vi "Change Selection.vi"(8 "error in (no error)":errorcluster, 10 "Coords":T1, 11 "PieChart in":refnum<class "PieChart.lvclass">) -> (0 "error out":errorcluster, 3 "PieChart out":refnum<class "PieChart.lvclass">)   [LabVIEW 2018, in "PieChart.lvclass"]
uses:
  PieChart.lvclass
  <vilib>/Utility/miscctls.llb/LVPoint32TypeDef.ctl
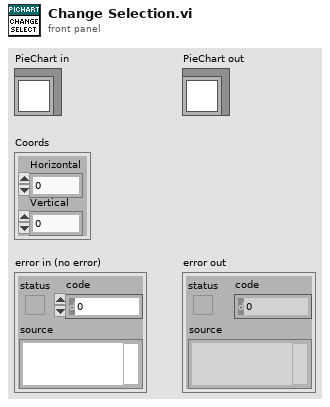
[diagram p1: front panel]
types:
  T1 = typedef "LVPoint32TypeDef.ctl" = cluster{"Horizontal":i32, "Vertical":i32}
  T2 = typedef "PieChart.lvclass/Pie info for Click.ctl" = cluster{"Slice Positions":cluster{"Start":i16, "End":i16}[], "Center Position":T3, "Radius":i16}
  T3 = typedef "LVBoundsTypeDef.ctl" = cluster{"Width":u32, "Height":u32}
  T4 = typedef "LVRectTypeDef.ctl" = cluster{"Left":i16, "Top":i16, "Right":i16, "Bottom":i16}
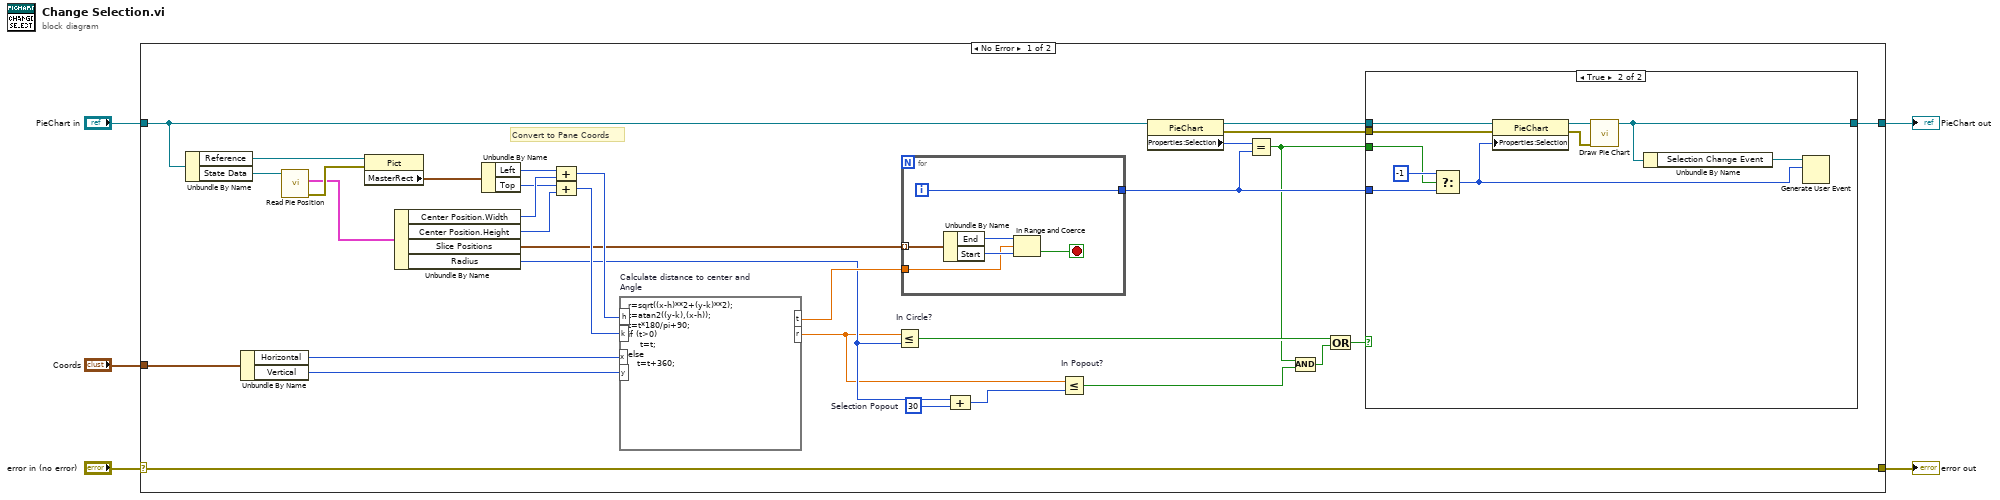
[diagram p0: block diagram]
diagram:
  n1 = case shown="No Error" "error in (no error)" {
    selector: "error in (no error)" -> [w37 w56]
    tunnel: [w37 w56] -> w4
    tunnel: [w20 w55] -> w2
    tunnel: "PieChart in" -> [w9 w55]
    tunnel: "Coords" -> [w27 _]
    frame No Error {
      w19 = i16 30  # Selection Popout
      # "Convert to Pane Coords"
      n2 = Unbundle By Name(w9) -> ("Reference"=w35:refnum<vi>, "State Data"=w36:refnum<data-value>)
      n3 = Unbundle By Name(w27) -> ("Horizontal"=w26:i32, "Vertical"=w25:i32)
      n4 = call "Read Pie Position.vi"("Data Value Reference in"=w36) -> ("error out"=w33:errorcluster, "Slice Positions"=w28:T2)  [unwired: 9 in]
      n5 = property class="Pict"(reference=w35, error in=w33) -> ("MasterRect"=w34:T4)  [unwired: 2 out]
      n6 = Unbundle By Name(w28) -> ("Center Position.Width"=w31:u32, "Center Position.Height"=w29:u32, "Slice Positions"=w6:cluster{"Start":i16, "End":i16}[], "Radius"=w18:i16)
      n7 = Unbundle By Name(w34) -> ("Left"=w32:i16, "Top"=w30:i16)
      n8 = Compound Arithmetic op=ADD(w32, w31) -> (w24:u32)
      n9 = Compound Arithmetic op=ADD(w30, w29) -> (w23:u32)
      n10 = formula code="r=sqrt((x-h)**2+(y-k)**2);\nt=atan2((y-k),(x-h));\nt=t*180/pi+90;\nif (t>0)\n    t=t;\nelse\n   t=t+360;" "Calculate distance to center and\nAngle"("x"=w26, "y"=w25, "h"=w24, "k"=w23) -> ("r"=w17:dbl, "t"=w22:dbl)
      n11 = Less Or Equal? "In Circle?"(x=w17, y=w18) -> (x <= y?=w15:bool)
      n12 = for {
        tunnel: w6 -> [w54] mode=indexing
        tunnel: w22 -> [w51]
        tunnel: [w49] -> w21
        i -> [w49]
        stop <- w50 stop-if-true
        n13 = Unbundle By Name(w54) -> ("End"=w52:i16, "Start"=w53:i16)
        n14 = In Range and Coerce(upper limit=w52, x=w51, lower limit=w53) -> (In Range?=w50:bool)  [unwired: 1 out]
      }
      n15 = Compound Arithmetic op=ADD(w18, w19) -> (w11:i16)
      n16 = Less Or Equal? "In Popout?"(x=w17, y=w11) -> (x <= y?=w12:bool)
      n17 = property class="PieChart"(reference=w9) -> (reference out=w8:refnum<class "PieChart.lvclass">, error out=w7:errorcluster, "Properties:Selection"=w14:i32)  [unwired: 1 in]
      n18 = Equal?(x=w14, y=w21) -> (x = y?=w13:bool)
      n19 = Compound Arithmetic op=AND(w13, w12) -> (w10:bool)
      n20 = Compound Arithmetic op=OR(w15, w10) -> (w16:bool)
      n21 = case shown="True" w16 {
        tunnel: w8 -> [w38 w46]
        tunnel: w21 -> [_ w44]
        tunnel: [w38 w41] -> w20
        tunnel: w13 -> [_ w43]
        tunnel: w7 -> [_ w42]
        frame False {
        }
        frame True {
          n22 = Select(t=-1, s=w43, f=w44) -> (s? t:f=w39:i32)
          n23 = property class="PieChart"(reference=w46, error in=w42, "Properties:Selection"=w39) -> (reference out=w48:refnum<class "PieChart.lvclass">, error out=w47:errorcluster)
          n24 = call-dynamic "Draw Pie Chart.vi"("error in (no error)"=w47, "PieChart in"=w48) -> ("PieChart out"=w41:refnum<class "PieChart.lvclass">)  [unwired: 8 in, 1 out]
          n25 = Unbundle By Name(w41) -> ("Selection Change Event"=w40:refnum<user-event>)
          n26 = Generate User Event(user event=w40, event data cluster=w39) -> ()  [unwired: 2 in, 2 out]
        }
      }
    }
    frame Error {
    }
  }
  "error out" <- w4
  "PieChart out" <- w2
